vi "PoissonRegressor.vi"(8 "error in":errorcluster) -> (0 "error out":errorcluster, 3 "out":refnum<class "PoissonRegressor.lvclass">)   [LabVIEW 2020]
doc: "Generalized Linear Model with a Poisson distribution.\n\n This regressor uses the 'log' link function.\n\n Read more in the :ref:`User Guide <Generalized_linear_regression>`.\n\n .. versionadded:: 0.23\n\n Parameters\n ----------\n alpha : float, default=1\n Constant that multiplies the penalty term and thus determines the\n regularization strength. ``alpha = 0`` is equivalent to unpenalized\n GLMs. In this case, the design matrix `X` must have full column rank\n (no collinearities).\n\n fit_intercept : bool, default=True\n Specifies if a constant (a.k.a. bias or intercept) should be\n added to the linear predictor (X @ coef + intercept).\n\n max_iter : int, default=100\n The maximal number of iterations for the solver.\n\n tol : float, default=1e-4\n Stopping criterion. For the lbfgs solver,\n the iteration will stop when ``max{|g_j|, j = 1, ..., d} <= tol``\n where ``g_j`` is the j-th component of the gradient (derivative) of\n the objective function.\n\n warm_start : bool, default=False\n If set to ``True``, reuse the solution of the previous call to ``fit``\n as initialization for ``coef_`` and ``intercept_`` .\n\n verbose : int, default=0\n For the lbfgs solver set verbose to any positive number for verbosity.\n\n Attributes\n ----------\n coef_ : array of shape (n_features,)\n Estimated coefficients for the linear predictor (`X @ coef_ +\n intercept_`) in the GLM.\n\n intercept_ : float\n Intercept (a.k.a. bias) added to linear predictor.\n\n n_iter_ : int\n Actual number of iterations used in the solver.\n\n \nAvailable methods:\nGet Attributes\nGet Params\nSet Params"
uses:
  PoissonRegressor.lvclass
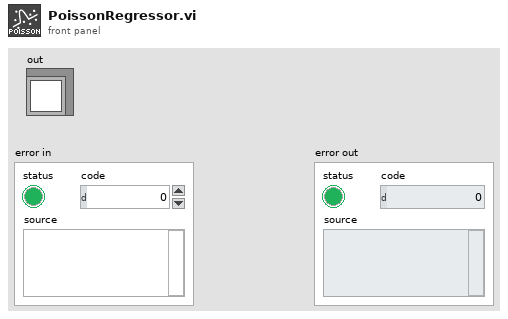
[diagram p1: front panel]
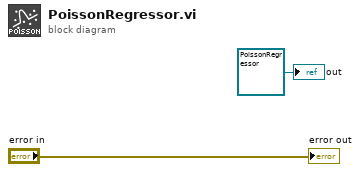
[diagram p0: block diagram]
diagram:
  "out" <- refnum<class "PoissonRegressor.lvclass"> refnum ("model")
  "error out" <- "error in"
